vi "Configure Operation Mode.vi"(8 "error in (no error)":errorcluster, 9 "Range (15)":dbl=15.0001 min=0.0001 max=7500.0 step=1.0 format="%.2f", 10 "Operation Mode (0:CC)":u16(ring) items=["CC", "CV", "CR", "CW"], 11 "VISA resource name":refnum<visa-resource-name>) -> (0 "error out":errorcluster, 3 "VISA resource name out":refnum<visa-resource-name>)   [LabVIEW 2020, in "BK Precision 8600 Series.lvlib"]
doc: "Configures the operation mode, range (for CC and CV mode), and setting limits (for CR, CW mode)."
uses:
  BK Precision 8600 Series.lvlib
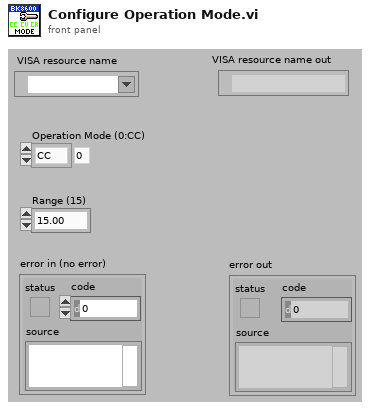
[diagram p1: front panel]
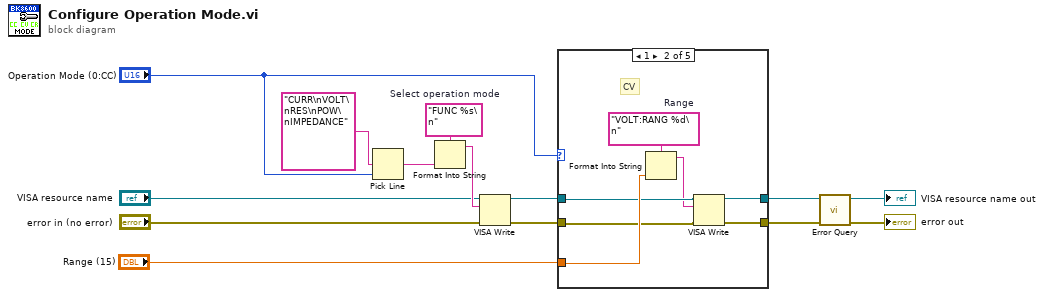
[diagram p0: block diagram]
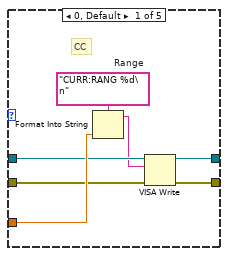
[diagram p2: hidden frame]
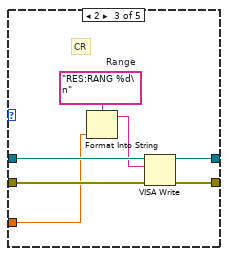
[diagram p3: hidden frame]
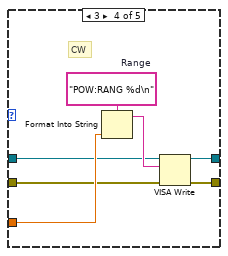
[diagram p4: hidden frame]
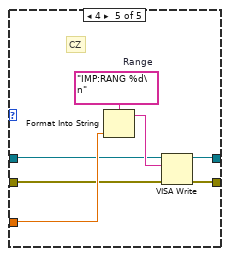
[diagram p5: hidden frame]
diagram:
  w12 = "FUNC %s\n"  # Select operation mode
  n1 = Pick Line(multi-line string="CURR\nVOLT\nRES\nPOW\nIMPEDANCE", line index="Operation Mode (0:CC)") -> (output string=w9:string)  [unwired: 1 in]
  n2 = Format Into String(format string=w12, w9) -> (resulting string=w11:string)  [unwired: 2 in, 1 out]
  n3 = VISA Write(VISA resource name="VISA resource name", write buffer=w11, error in (no error)="error in (no error)") -> (VISA resource name out=w6:refnum<visa-resource-name>, error out=w7:errorcluster)  [unwired: 1 out]
  n4 = case shown="1" "Operation Mode (0:CC)" {
    tunnel: w7 -> [w16 w24 w35 w39 w46]
    tunnel: w6 -> [w17 w23 w34 w38 w45]
    tunnel: [w21 w28 w33 w37 w44] -> w5
    tunnel: [w20 w27 w32 w36 w43] -> w4
    tunnel: "Range (15)" -> [w18 w25 w29 w40 w47]
    frame 0, Default {
      w19 = "CURR:RANG %d\n"  # Range
      # "CC"
      n5 = Format Into String(format string=w19, w18) -> (resulting string=w15:string)  [unwired: 2 in, 1 out]
      n6 = VISA Write(VISA resource name=w17, write buffer=w15, error in (no error)=w16) -> (VISA resource name out=w21:refnum<visa-resource-name>, error out=w20:errorcluster)  [unwired: 1 out]
    }
    frame 1 {
      w26 = "VOLT:RANG %d\n"  # Range
      # "CV"
      n7 = Format Into String(format string=w26, w25) -> (resulting string=w22:string)  [unwired: 2 in, 1 out]
      n8 = VISA Write(VISA resource name=w23, write buffer=w22, error in (no error)=w24) -> (VISA resource name out=w28:refnum<visa-resource-name>, error out=w27:errorcluster)  [unwired: 1 out]
    }
    frame 2 {
      w31 = "RES:RANG %d\n"  # Range
      # "CR"
      n9 = Format Into String(format string=w31, w29) -> (resulting string=w30:string)  [unwired: 2 in, 1 out]
      n10 = VISA Write(VISA resource name=w34, write buffer=w30, error in (no error)=w35) -> (VISA resource name out=w33:refnum<visa-resource-name>, error out=w32:errorcluster)  [unwired: 1 out]
    }
    frame 3 {
      w42 = "POW:RANG %d\n"  # Range
      # "CW"
      n11 = Format Into String(format string=w42, w40) -> (resulting string=w41:string)  [unwired: 2 in, 1 out]
      n12 = VISA Write(VISA resource name=w38, write buffer=w41, error in (no error)=w39) -> (VISA resource name out=w37:refnum<visa-resource-name>, error out=w36:errorcluster)  [unwired: 1 out]
    }
    frame 4 {
      w49 = "IMP:RANG %d\n"  # Range
      # "CZ"
      n13 = Format Into String(format string=w49, w47) -> (resulting string=w48:string)  [unwired: 2 in, 1 out]
      n14 = VISA Write(VISA resource name=w45, write buffer=w48, error in (no error)=w46) -> (VISA resource name out=w44:refnum<visa-resource-name>, error out=w43:errorcluster)  [unwired: 1 out]
    }
  }
  n15 = call "Error Query.vi"("error in (no error)"=w4, "VISA resource name"=w5) -> ("error out"=→"error out":errorcluster, "VISA resource name out"=→"VISA resource name out":refnum<visa-resource-name>)  [unwired: 6 in, 2 out]
